vi "TempFileLoad.vi"(9 "거리 해상도":sgl, 10 "온도 데이터 경로 문자열":string) -> (0 "온도 인덱스":i32 caption="스톡스 인덱스", 2 "온도 배열":dbl[](array[numeric]) caption="온도 데이터 배열", 4 "거리축 배열":dbl[](array[numeric]), 6 "대기중":bool)   [LabVIEW 2020]
uses:
  <vilib>/Utility/error.llb/DialogType.ctl
panel:
  out "스톡스 읽기 완료":bool caption="읽기완료"
  out "온도 데이터 경로":path
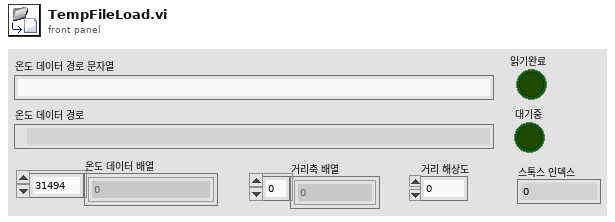
[diagram p1: front panel]
types:
  T1 = typedef "DialogType.ctl" = u16
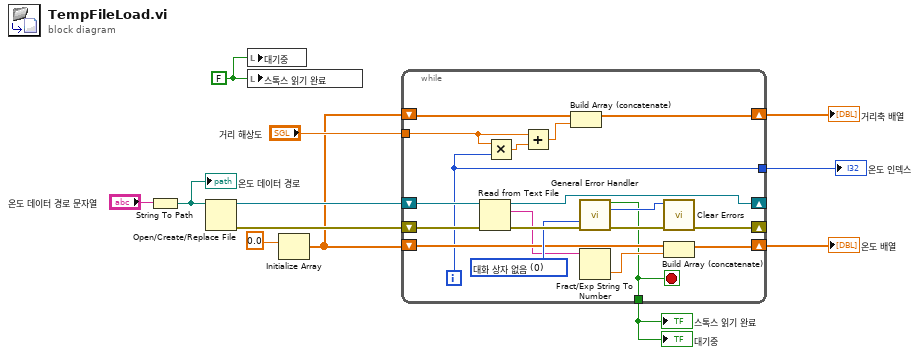
[diagram p0: block diagram]
diagram:
  w2 = FALSE
  n1 = String To Path(string="온도 데이터 경로 문자열") -> (path=w10:path)
  "온도 데이터 경로" <- w10
  n2 = Open/Create/Replace File(file path (use dialog)=w10) -> (refnum out=w12:refnum<file>, error out=w11:errorcluster)  [unwired: 5 in, 1 out]
  n3 = local write "대기중"(w2) -> ()
  n4 = local write "스톡스 읽기 완료"(w2) -> ()
  n5 = Initialize Array(0.0) -> (w4:dbl[])  [unwired: 1 in]
  n6 = while {
    shift-right: [w26] -> _
    shift-left: w12 -> [w31]
    shift-right: [w27] -> _
    shift-left: w11 -> [w30]
    tunnel: [w14] -> w8
    shift-right: [w22] -> w6
    shift-left: w4 -> [w23]
    tunnel: "거리 해상도" -> [w19]
    shift-right: [w16] -> w3
    shift-left: w4 -> [w18]
    tunnel: [w13] -> w1
    i -> [w13]
    stop <- w14 stop-if-true
    w24 = T1 0 items=["대화 상자 없음", "확인 메시지", "메시지 지속 또는 정지", "확인 메시지 + 경고", "지속/정지 + 경고"] ("type of dialog (OK msg:1)")
    n7 = Read from Text File(file (use dialog)=w31, error in=w30) -> (refnum out=w26:refnum<file>, text=w21:string, error out=w28:errorcluster)  [unwired: 2 in, 1 out]
    n8 = Multiply(x=w19, y=w13) -> (x*y=w20:sgl)
    n9 = Add(x=w19, y=w20) -> (x+y=w17:sgl)
    n10 = Build Array (concatenate)(w18, w17) -> (w16:dbl[])
    n11 = call <vilib>:"General Error Handler.vi"("type of dialog (OK msg:1)"=w24, "error in (no error)"=w28) -> ("error?"=w14:bool, "code out"=w29:i32, "error out"=w25:errorcluster)  [unwired: 9 in, 2 out]
    n12 = Fract/Exp String To Number(string=w21) -> (number=w15:dbl)  [unwired: 3 in, 1 out]
    n13 = call <vilib>:"Clear Errors.vi"("error in (no error)"=w25, "specific error code to clear (0: all)"=w29) -> ("error out"=w27:errorcluster)  [unwired: 4 in, 1 out]
    n14 = Build Array (concatenate)(w23, w15) -> (w22:dbl[])
  }
  "대기중" <- w8
  "스톡스 읽기 완료" <- w8
  "온도 배열" <- w6
  "온도 인덱스" <- w1
  "거리축 배열" <- w3
